vi "Rocket.vi"() -> ()   [LabVIEW 2014]
uses:
  Control 1.ctl
panel:
  out "Timeout State":bool
  out "Abort State":bool
  out "Engine Stop":bool
  out "Countdown State":bool
  out "Fire State":bool
  out "Ready State":bool
  in  "?":bool
  out "Count":dbl
  in  "?":bool
  out "Engine":bool
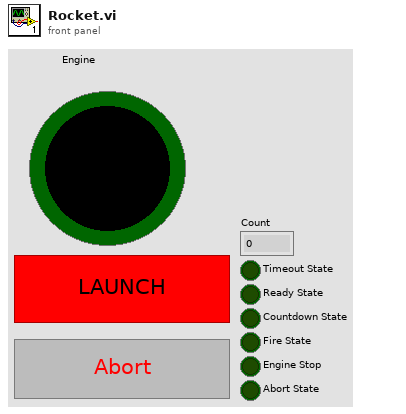
[diagram p1: front panel]
types:
  T1 = typedef "Control 1.ctl" = enum16{"Timeout", "Ready", "Countdown", "Fire", "Engine Stop", "Abort"}
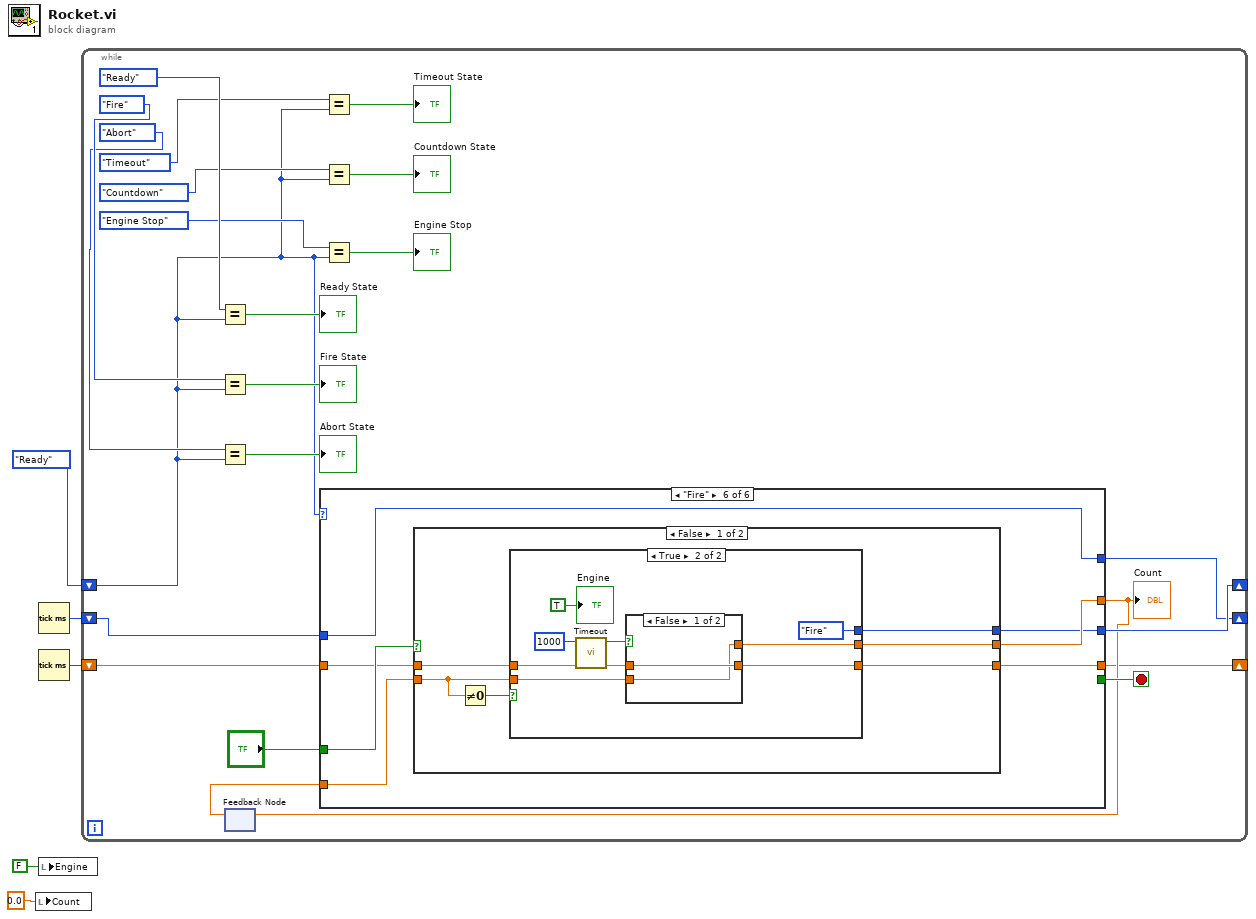
[diagram p0: block diagram]
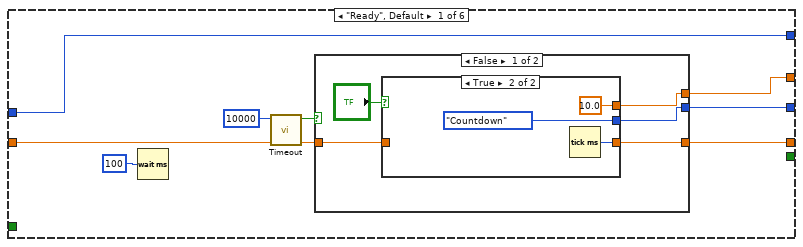
[diagram p2: hidden frame]
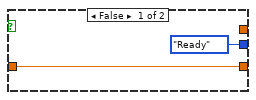
[diagram p3: hidden frame]
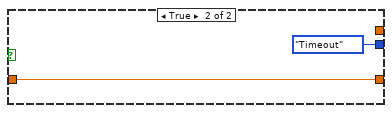
[diagram p4: hidden frame]
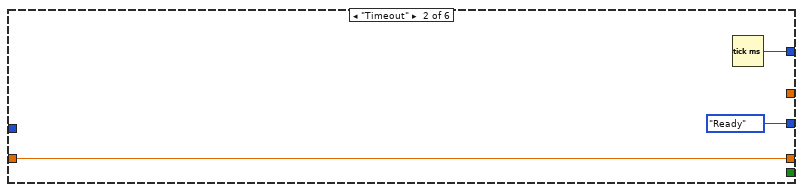
[diagram p5: hidden frame]
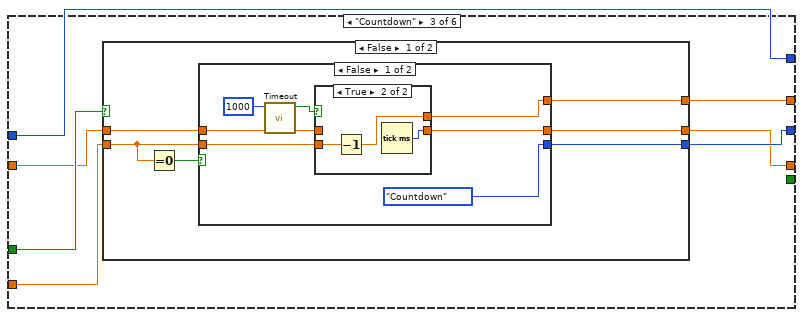
[diagram p6: hidden frame]
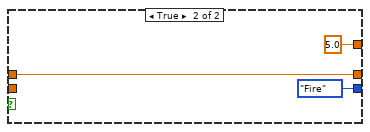
[diagram p8: hidden frame]
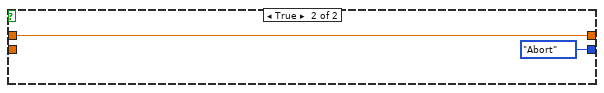
[diagram p9: hidden frame]
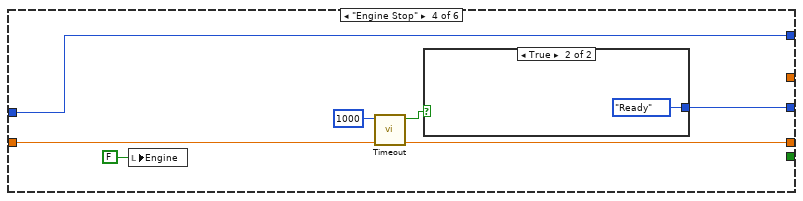
[diagram p10: hidden frame]
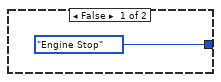
[diagram p11: hidden frame]
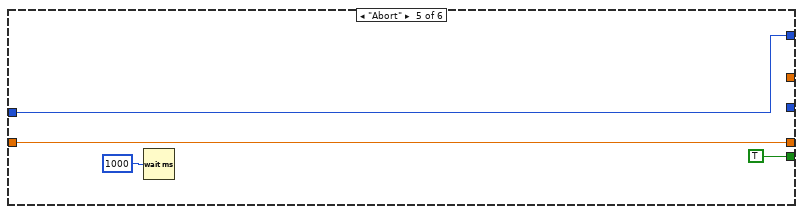
[diagram p12: hidden frame]
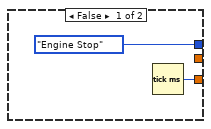
[diagram p13: hidden frame]
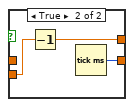
[diagram p14: hidden frame]
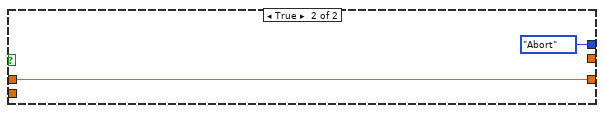
[diagram p15: hidden frame]
diagram:
  n1 = local write "Count"(0.0) -> ()
  n2 = Tick Count (ms)() -> (millisecond timer value=w2:u32)
  n3 = Tick Count (ms)() -> (millisecond timer value=w1:u32)
  n4 = local write "Engine"(FALSE) -> ()
  n5 = while {
    shift-right: [w26] -> _
    shift-left: Control_1."Ready" ("Launch State") -> [w10]
    shift-right: [w8] -> _
    shift-left: w2 -> [w9]
    shift-right: [w6] -> _
    shift-left: w1 -> [w7]
    stop <- w25 stop-if-true
    n6 = Equal?(x=Control_1."Ready" ("Launcher State"), y=w10) -> (x = y?=→"Ready State":bool)
    n7 = Equal?(x=Control_1."Fire" ("Launcher State"), y=w10) -> (x = y?=→"Fire State":bool)
    n8 = Equal?(x=Control_1."Abort" ("Launcher State"), y=w10) -> (x = y?=→"Abort State":bool)
    n9 = feedback #1() -> (w24:dbl)  [unwired: 1 in]
    n10 = case shown="\"Fire\"" w10 {
      tunnel: "?" -> [_ _ w58 _ _ w102]
      tunnel: [w36 _ w57 _ _ w101] -> w23
      tunnel: w24 -> [_ _ w56 _ _ w100]
      tunnel: [w35 Control_1."Ready" ("Launcher State") w55 w87 _ w99] -> w26
      tunnel: [_ _ _ _ TRUE _] -> w25
      tunnel: w9 -> [w30 _ w54 w88 w93 w98]
      tunnel: [w30 w50 w54 w88 w93 w98] -> w8
      tunnel: w7 -> [w29 w49 w53 w83 w92 w96]
      tunnel: [w32 w49 w52 w86 w92 w97] -> w6
      frame "Ready", Default {
        n11 = Wait (ms)(milliseconds to wait=100) -> ()  [unwired: 1 out]
        n12 = call "Timeout.vi"("Start Time In"=w29, "Limit In"=10000) -> ("Start Time Out"=w28:dbl, "Timeout"=w33:bool)  [unwired: 8 in]
        n13 = case shown="False" w33 {
          tunnel: [w41 _] -> w36
          tunnel: [w40 Control_1."Timeout" ("Launch State")] -> w35
          tunnel: [w38 w47] -> w32
          tunnel: w28 -> [w37 w47]
          frame False {
            n14 = case shown="True" "?" {
              tunnel: [_ 10.0 ("Count")] -> w41
              tunnel: [Control_1."Ready" ("Launch State") Control_1."Countdown" ("Launch State")] -> w40
              tunnel: [w42 w44] -> w38
              tunnel: w37 -> [w42 _]
              frame False {
              }
              frame True {
                n15 = Tick Count (ms)() -> (millisecond timer value=w44:u32)
              }
            }
          }
          frame True {
          }
        }
      }
      frame "Timeout" {
        n16 = Tick Count (ms)() -> (millisecond timer value=w50:u32)
      }
      frame "Countdown" {
        n17 = case shown="False" w58 {
          tunnel: [w64 _] -> w57
          tunnel: w56 -> [w63 _]
          tunnel: [w61 Control_1."Abort" ("Launch State")] -> w55
          tunnel: w53 -> [w60 w81]
          tunnel: [w59 w81] -> w52
          frame False {
            n18 = Equal To 0?(x=w63) -> (x = 0?=w62:bool)
            n19 = case shown="False" w62 {
              tunnel: [w70 5.0 ("Count")] -> w64
              tunnel: w63 -> [w68 _]
              tunnel: [Control_1."Countdown" ("Launch State") Control_1."Fire" ("Launch State")] -> w61
              tunnel: w60 -> [w67 w78]
              tunnel: [w65 w78] -> w59
              frame False {
                n20 = call "Timeout.vi"("Start Time In"=w67, "Limit In"=1000) -> ("Start Time Out"=w66:dbl, "Timeout"=w71:bool)  [unwired: 8 in]
                n21 = case shown="True" w71 {
                  tunnel: w68 -> [w74 w77]
                  tunnel: [w74 w76] -> w70
                  tunnel: w66 -> [w73 _]
                  tunnel: [w73 w75] -> w65
                  frame False {
                  }
                  frame True {
                    n22 = Decrement(x=w77) -> (x-1=w76:dbl)
                    n23 = Tick Count (ms)() -> (millisecond timer value=w75:u32)
                  }
                }
              }
              frame True {
              }
            }
          }
          frame True {
          }
        }
      }
      frame "Engine Stop" {
        n24 = local write "Engine"(FALSE) -> ()
        n25 = call "Timeout.vi"("Start Time In"=w83, "Limit In"=u32 1000 ("millisecond timer value")) -> ("Start Time Out"=w86:dbl, "Timeout"=w85:bool)  [unwired: 8 in]
        n26 = case shown="True" w85 {
          tunnel: [Control_1."Engine Stop" ("Launch State") Control_1."Ready" ("Launch State")] -> w87
          frame False {
          }
          frame True {
          }
        }
      }
      frame "Abort" {
        n27 = Wait (ms)(milliseconds to wait=u32 1000 ("millisecond timer value")) -> ()  [unwired: 1 out]
      }
      frame "Fire" {
        n28 = case shown="False" w102 {
          tunnel: [w108 _] -> w101
          tunnel: [w107 Control_1."Abort" ("Launch State")] -> w99
          tunnel: w100 -> [w106 _]
          tunnel: [w104 w125] -> w97
          tunnel: w96 -> [w103 w125]
          frame False {
            n29 = Not Equal To 0?(x=w106) -> (x != 0?=w105:bool)
            n30 = case shown="True" w105 {
              tunnel: [_ w113] -> w108
              tunnel: [Control_1."Engine Stop" ("Launch State") Control_1."Fire" ("Launcher State")] -> w107
              tunnel: w106 -> [_ w114]
              tunnel: [w109 w112] -> w104
              tunnel: w103 -> [_ w117]
              frame False {
                n31 = Tick Count (ms)() -> (millisecond timer value=w109:u32)
              }
              frame True {
                n32 = call "Timeout.vi"("Start Time In"=w117, "Limit In"=1000) -> ("Start Time Out"=w115:dbl, "Timeout"=w111:bool)  [unwired: 8 in]
                n33 = case shown="False" w111 {
                  tunnel: [w121 w124] -> w112
                  tunnel: w115 -> [w121 _]
                  tunnel: w114 -> [w120 w123]
                  tunnel: [w120 w122] -> w113
                  frame False {
                  }
                  frame True {
                    n34 = Decrement(x=w123) -> (x-1=w122:dbl)
                    n35 = Tick Count (ms)() -> (millisecond timer value=w124:u32)
                  }
                }
                "Engine" <- TRUE
              }
            }
          }
          frame True {
          }
        }
      }
    }
    "Count" <- w23
    n36 = feedback-in #1(w23) -> ()
    n37 = Equal?(x=Control_1."Timeout" ("Launcher State"), y=w10) -> (x = y?=→"Timeout State":bool)
    n38 = Equal?(x=Control_1."Countdown" ("Launcher State"), y=w10) -> (x = y?=→"Countdown State":bool)
    n39 = Equal?(x=Control_1."Engine Stop" ("Launcher State"), y=w10) -> (x = y?=→"Engine Stop":bool)
  }
